vi "Main.vi"(11 "Module Admin":refnum<class "Delacor_lib_QMH_Module Admin.lvclass">) -> ()   [LabVIEW 2020, in "Aqcisition.lvlib"]
doc: "This template is based off of the Queued Message Handler design pattern and the Queued Message Handler project template that ships with LabVIEW.\n\nThe main difference is that the queue is private to this module and communication between modules is performed via Broadcast and Request events.\n\nRequest events are wrapped in public API methods and are handled in the Event Handling Loop (EHL) of this VI. Any module can register for Broadcast events sent by this module. The EHL generates messages based on user interface actions.\n\nThe Message Handling Loop (MHL) processes messages generated by the EHL, or by other messages. The messages are string values, so new messages can be added easily to the Message Cases case structure in the MHL. Each message cluster can also provide an optional value for Message Data, which is a variant that can be converted to whatever message-specific data is required.\n_____\nBased on Delacor QMH Project Template 6.0.0.89."
uses:
  Aqcisition.lvlib
  <vilib>/Delacor/Delacor QMH/Libraries/Module Admin_class/Delacor_lib_QMH_Module Admin.lvclass
  Module Data--cluster.ctl
  Analog Signal Config.ctl
  Digital Signal Config.ctl
  Stop Argument--cluster.ctl
  <vilib>/Delacor/Delacor QMH/Libraries/Message Queue_class/Delacor_lib_QMH_Message Queue.lvclass/Delacor_lib_QMH_Message Queue.ctl
  <vilib>/Delacor/Delacor QMH/Libraries/Module Admin_class/Delacor_lib_QMH_Module Admin.lvclass/Delacor_lib_QMH_Module Admin.ctl
  Start Adqcisition Argument--cluster.ctl
  Stop Adqcisition Argument--cluster.ctl
  Set AQ Parameters Argument--cluster.ctl
  <vilib>/Utility/miscctls.llb/LVPointTypeDef.ctl
  <vilib>/DAQmx/read.llb/DAQmx Read (Digital 1D U8 NChan 1Samp).vi
  <vilib>/DAQmx/read.llb/DAQmx Read (Analog 1D Wfm NChan NSamp).vi
  <vilib>/Delacor/Delacor QMH/Libraries/Message Queue_class/Delacor_lib_QMH_Enqueue Message (Single).vi
  <vilib>/Delacor/Delacor QMH/Libraries/Module Admin_class/Delacor_lib_QMH_Get External Launch.vi
  <vilib>/DAQmx/miscellaneous.llb/DAQmx Fill In Error Info.vi
  <vilib>/Utility/error.llb/Error Cluster From Error Code.vi
  <vilib>/ErrorRing/Error Ring.xnode
  <vilib>/Delacor/Delacor QMH/Libraries/Message Queue_class/Delacor_lib_QMH_Message Queue.lvclass
panel:
  out "error out":errorcluster
  out "Status":string
types:
  T1 = typedef "Aqcisition.lvlib/Request Events--cluster.ctl" = cluster{"Stop Module":refnum<user-event>, "Show Panel":refnum<user-event>, "Hide Panel":refnum<user-event>, "Get Module Execution Status":refnum<user-event>, "Show Diagram":refnum<user-event>, "Start Adqcisition":refnum<user-event>, "Stop Adqcisition":refnum<user-event>, "Wake Up Helper Loop":refnum<user-event>, "Put HL to Sleep":refnum<user-event>, "Set AQ Parameters":refnum<user-event>, "Wake up Digital Loop":refnum<user-event>}
  T2 = typedef "Aqcisition.lvlib/Module Data--cluster.ctl" = cluster{"Status":string, "Señal Analogica":T3, "Señal Digital":T4}
  T3 = typedef "Analog Signal Config.ctl" = cluster{"Canal/Canales":string, "Canal":tag, "Canales":tag[], "Frecuencia de muestreo":i32, "Numero de muestras":i32, "Tiempo de AQ":dbl}
  T4 = typedef "Digital Signal Config.ctl" = cluster{"Puertos/Pines":string, "Puerto":tag, "Pines":tag[], "Tiempo de AQ":dbl, "Tiempo entre AQ":dbl}
  T5 = enum32{"invalid lock state", "Not Locked", "Locked (No Password)", "Password-protected"}
  T6 = typedef "Aqcisition.lvlib/Stop Argument--cluster.ctl" = cluster{"Origin":string, "Exit via Stop Module Req?":bool, "Wait for Module to stop?":bool}
  T7 = typedef "Aqcisition.lvlib/Start Adqcisition Argument--cluster.ctl" = cluster{"Boolean":bool}
  T8 = typedef "Aqcisition.lvlib/Stop Adqcisition Argument--cluster.ctl" = cluster{"Boolean":bool}
  T9 = typedef "Aqcisition.lvlib/Set AQ Parameters Argument--cluster.ctl" = cluster{"Señal Analogica":T3, "Señal Digital":T4}
  T10 = typedef "LVPointTypeDef.ctl" = cluster{"Horizontal":i16, "Vertical":i16}
  T11 = enum32{"Invalid", "Standard", "Closed", "Hidden", "Minimized", "Maximized"}
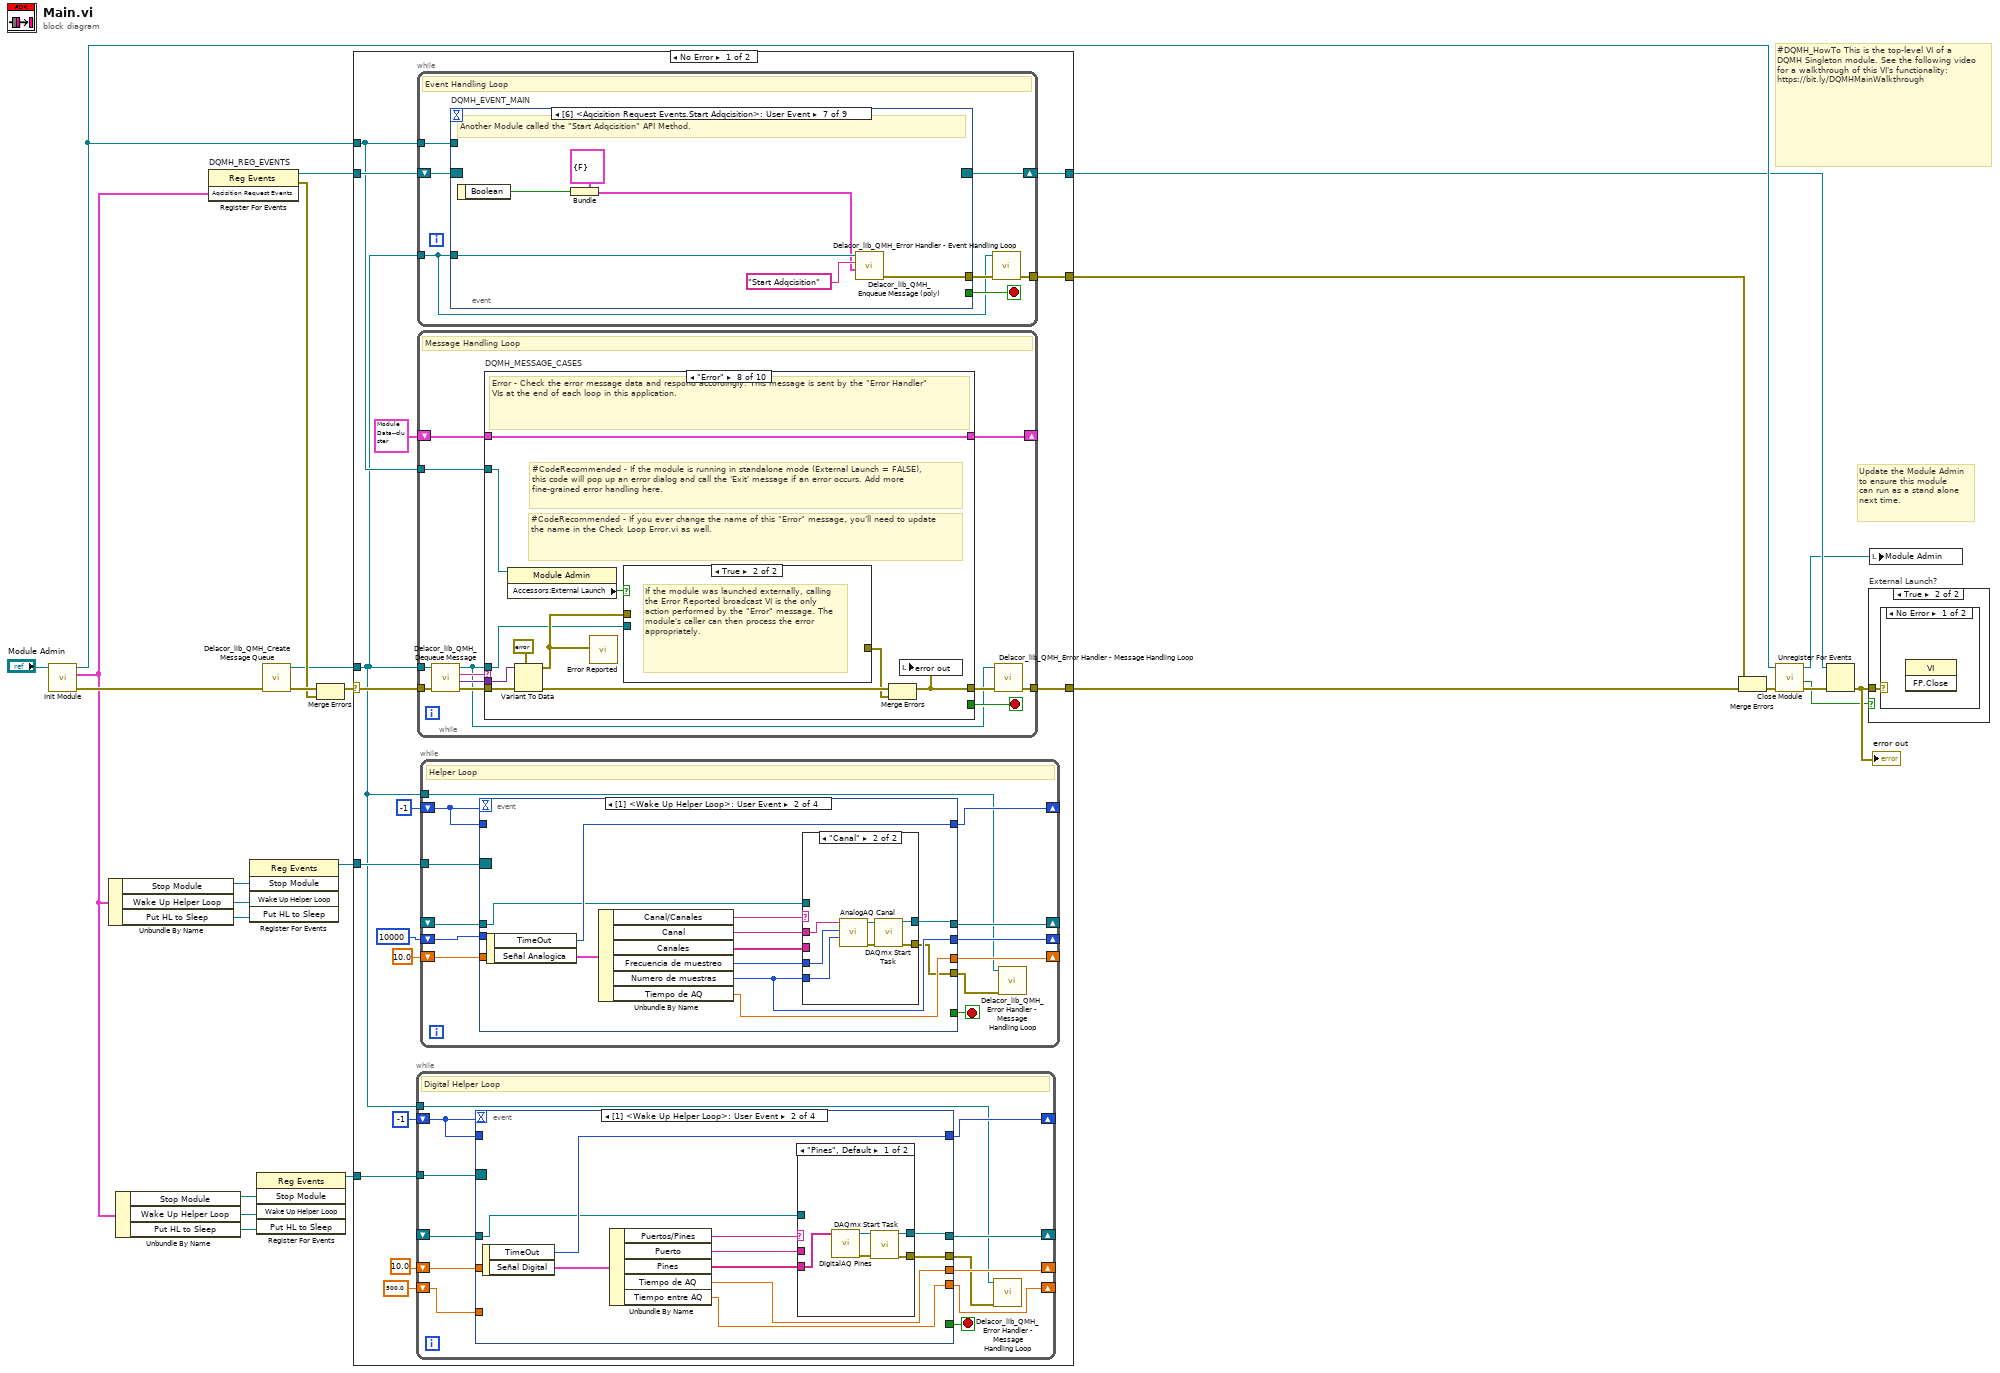
[diagram p0: block diagram]
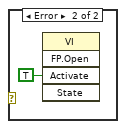
[diagram p3: hidden frame]
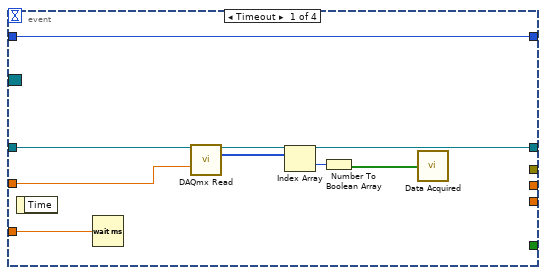
[diagram p4: hidden frame]
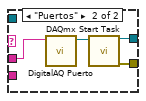
[diagram p5: hidden frame]
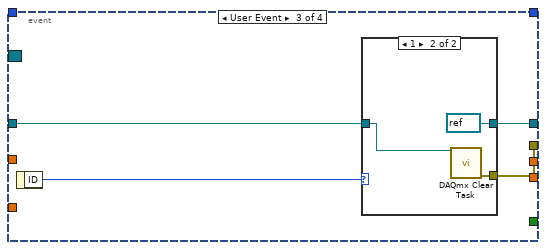
[diagram p6: hidden frame]
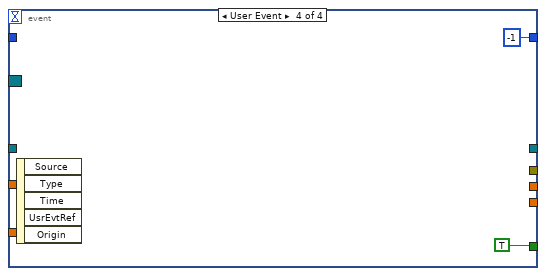
[diagram p8: hidden frame]
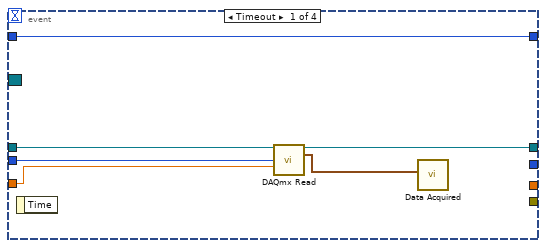
[diagram p9: hidden frame]
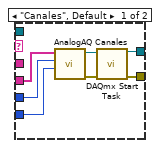
[diagram p10: hidden frame]
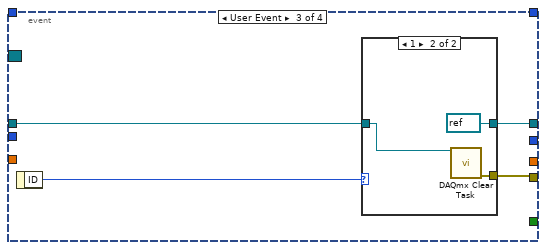
[diagram p11: hidden frame]
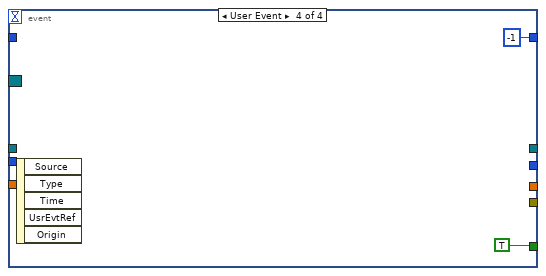
[diagram p13: hidden frame]
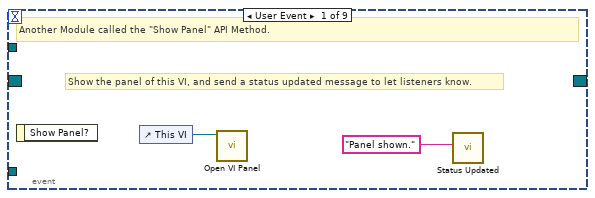
[diagram p14: hidden frame]
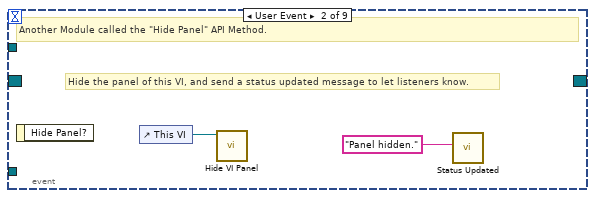
[diagram p15: hidden frame]
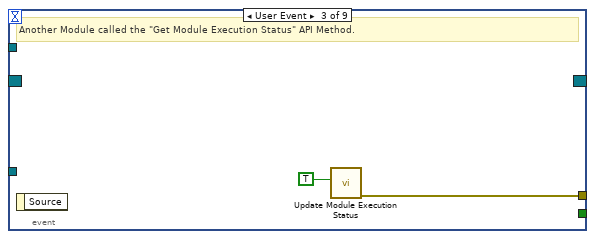
[diagram p16: hidden frame]
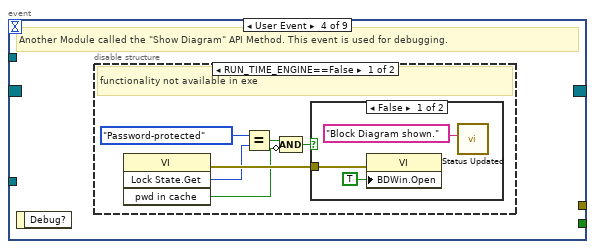
[diagram p17: hidden frame]
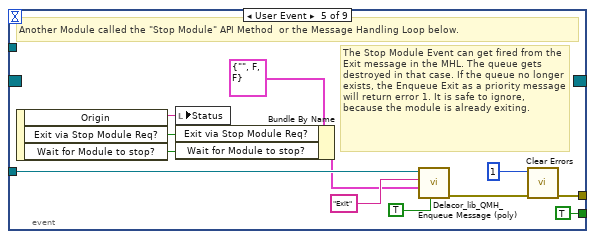
[diagram p20: hidden frame]
diagram:
  # "#DQMH_HowTo This is the top-level VI of a DQMH Singleton module. See the following video for a walkthrough of this VI's functionality: https://bit.ly/DQMHMainWalkthrough"
  # "Update the Module Admin to ensure this module can run as a stand alone next time."
  n1 = call "Init Module.vi"("Singleton Module Admin in"="Module Admin") -> ("error out"=w24:errorcluster, "Aqcisition Request Events"=w2:T1, "Singleton Module Admin out"=w16:refnum<class "Delacor_lib_QMH_Module Admin.lvclass">)  [unwired: 8 in]
  n2 = Unbundle By Name(w2) -> ("Stop Module"=w8:refnum<user-event>, "Wake Up Helper Loop"=w7:refnum<user-event>, "Put HL to Sleep"=w6:refnum<user-event>)
  n3 = Unbundle By Name(w2) -> ("Stop Module"=w3:refnum<user-event>, "Wake Up Helper Loop"=w4:refnum<user-event>, "Put HL to Sleep"=w5:refnum<user-event>)
  n4 = register-events "DQMH_REG_EVENTS"(w2) -> (reference out=w14:refnum<event-registration>, error out=w17:errorcluster)  [unwired: 2 in]
  n5 = register-events(w8, w7, w6) -> (reference out=w9:refnum<event-registration>)  [unwired: 2 in, 1 out]
  n6 = register-events(w3, w4, w5) -> (reference out=w1:refnum<event-registration>)  [unwired: 2 in, 1 out]
  n7 = call <vilib>:"Delacor_lib_QMH_Create Message Queue.vi"("error in"=w24) -> ("error out"=w19:errorcluster, "Message Queue"=w13:refnum<class "Delacor_lib_QMH_Message Queue.lvclass">)  [unwired: 9 in]
  n8 = Merge Errors(w19, w17) -> (w18:errorcluster)
  n9 = case shown="No Error" w18 {
    selector: w18 -> [w39 w315]
    tunnel: [w41 w314] -> w25
    tunnel: [w38 w320] -> w15
    tunnel: w14 -> [w36 w320]
    tunnel: w13 -> [w30 w313]
    tunnel: [w40 _] -> w22
    tunnel: w16 -> [w31 w316]
    tunnel: w9 -> [w34 _]
    tunnel: w1 -> [w29 _]
    frame No Error {
      n10 = while {
        shift-right: [w52] -> _
        shift-left: -1 ("TimeOut") -> [w53]
        tunnel: w29 -> [w51]
        shift-right: [w49] -> _
        shift-left: _ -> [w50]
        shift-right: [w48] -> _
        shift-left: 10.0 -> [w47]
        tunnel: w30 -> [w44]
        shift-right: [w43] -> _
        shift-left: 500.0 ("Tiempo entre AQ") -> [w42]
        stop <- w46 stop-if-true
        # "Digital Helper Loop"
        n11 = event shown="[1] <Wake Up Helper Loop>: User Event" {
          selector: w51 -> [_ _ _ _]
          dyn-events: _ -> [_ _ _ _]
          timeout: w53 -> [_ _ _ _]
          tunnel: w53 -> [w61 _ _ _]
          tunnel: [w61 w71 _ -1 ("TimeOut")] -> w52
          tunnel: w50 -> [w60 w66 w84 _]
          tunnel: [w59 w65 w83 _] -> w49
          tunnel: [_ w63 _ _] -> w48
          tunnel: w47 -> [w58 _ _ _]
          tunnel: [_ _ _ TRUE] -> w46
          tunnel: [_ w64 w81 _] -> w45
          tunnel: [_ w62 _ _] -> w43
          tunnel: w42 -> [w54 _ _ _]
          event Timeout {
            n12 = event-data() -> ()  [unwired: 1 in, 1 out]
            n13 = Wait (ms)(milliseconds to wait=w54) -> ()  [unwired: 1 out]
            n14 = call-poly <vilib>:"DAQmx Read.vi"("task/channels in"=w60, "timeout"=w58) -> ("task out"=w59:refnum<k21>, "data"=w57:u8[])  [unwired: 11 in, 1 out]
            n15 = Index Array(array=w57) -> (element=w56:u8)  [unwired: 1 in]
            n16 = Number To Boolean Array(number=w56) -> (Boolean array=w55:bool[])
            n17 = call "Data Acquired.vi"("Digital"=w55) -> ()  [unwired: 10 in, 1 out]
          }
          event User Event {
            n18 = event-data() -> ("TimeOut"=w71:i32, "Señal Digital"=w70:T4)  [unwired: 1 in]
            n19 = Unbundle By Name(w70) -> ("Puertos/Pines"=w69:string, "Puerto"=w68:tag, "Pines"=w67:tag[], "Tiempo de AQ"=w63:dbl, "Tiempo entre AQ"=w62:dbl)
            n20 = case shown="\"Pines\", Default" w69 {
              tunnel: w68 -> [_ w78]
              tunnel: w67 -> [w72 _]
              tunnel: w66 -> [_ _]
              tunnel: [w76 w80] -> w65
              tunnel: [w75 w79] -> w64
              frame "Pines", Default {
                n21 = call "DigitalAQ Pines.vi"("Array"=w72) -> ("error out"=w73:errorcluster, "Classic DAQmx Task Name"=w74:refnum<k21>)  [unwired: 9 in]
                n22 = call <vilib>:"DAQmx Start Task.vi"("task/channels in"=w74, "error in"=w73) -> ("task out"=w76:refnum<k21>, "error out"=w75:errorcluster)  [unwired: 12 in]
              }
              frame "Puertos" {
                n23 = call "DigitalAQ Puerto.vi"("DAQmx Board Name"=w78) -> ("Classic DAQmx Task Name"=w77:refnum<k21>)  [unwired: 9 in, 1 out]
                n24 = call <vilib>:"DAQmx Start Task.vi"("task/channels in"=w77) -> ("task out"=w80:refnum<k21>, "error out"=w79:errorcluster)  [unwired: 13 in]
              }
            }
          }
          event User Event {
            n25 = event-data() -> ("ID"=w82:i32)  [unwired: 1 in]
            n26 = case shown="1" w82 {
              tunnel: w84 -> [w85 w88]
              tunnel: [w85 refnum<k21> refnum ("task out")] -> w83
              tunnel: [_ w86] -> w81
              frame 0, Default {
              }
              frame 1 {
                n27 = call <vilib>:"DAQmx Clear Task.vi"("task in"=w88) -> ("error out"=w86:errorcluster)  [unwired: 14 in]
              }
            }
          }
          event User Event {
            n28 = event-data() -> ()  [unwired: 1 in, 5 out]
          }
        }
        n29 = call-dynamic "Delacor_lib_QMH_Error Handler - Message Handling Loop.vi"("error in"=w45, "Message Queue in"=w44) -> ()  [unwired: 8 in, 2 out]
      }
      n30 = while {
        tunnel: w30 -> [w144]
        shift-right: [w147] -> w38
        shift-left: w36 -> [w148]
        tunnel: [w149] -> w40
        tunnel: w31 -> [w145]
        stop <- w146 stop-if-true
        # "Event Handling Loop"
        n31 = event "DQMH_EVENT_MAIN" shown="[6] <Aqcisition Request Events.Start Adqcisition>: User Event" {
          selector: w148 -> [_ _ _ _ _ _ _ _ _]
          dyn-events: [_ _ _ _ _ _ _ _ _] -> w147
          timeout: _ -> [_ _ _ _ _ _ _ _ _]
          tunnel: [_ _ _ _ TRUE ("Discard?") _ _ _ _] -> w146
          tunnel: w144 -> [_ _ _ _ w173 w180 w193 w199 w206]
          tunnel: [_ _ w156 _ w176 w182 w188 w194 w200] -> w150
          tunnel: w145 -> [_ _ _ _ _ w179 _ _ _]
          event User Event {
            # "Show the panel of this VI, and send a status updated message to let listeners know."
            # "Another Module called the \"Show Panel\" API Method."
            n32 = event-data() -> ()  [unwired: 1 in, 1 out]
            n33 = control-ref of="This VI"() -> (w152:refnum<vi>)
            n34 = call "Open VI Panel.vi"("VI"=w152) -> ()  [unwired: 10 in, 1 out]
            n35 = call "Status Updated.vi"("Status"="Panel shown." ("format string")) -> ()  [unwired: 10 in, 1 out]
          }
          event User Event {
            # "Hide the panel of this VI, and send a status updated message to let listeners know."
            # "Another Module called the \"Hide Panel\" API Method."
            n36 = event-data() -> ()  [unwired: 1 in, 1 out]
            n37 = control-ref of="This VI"() -> (w154:refnum<vi>)
            n38 = call "Hide VI Panel.vi"("VI"=w154) -> ()  [unwired: 10 in, 1 out]
            n39 = call "Status Updated.vi"("Status"="Panel hidden." ("format string")) -> ()  [unwired: 10 in, 1 out]
          }
          event User Event {
            # "Another Module called the \"Get Module Execution Status\" API Method."
            n40 = event-data() -> ()  [unwired: 1 in, 1 out]
            n41 = call "Update Module Execution Status.vi"("Running?"=TRUE) -> ("error out"=w156:errorcluster)  [unwired: 10 in]
          }
          event User Event {
            # "Another Module called the \"Show Diagram\" API Method. This event is used for debugging."
            n42 = event-data() -> ()  [unwired: 1 in, 1 out]
            n43 = disable-structure shown="RUN_TIME_ENGINE==False" {
              frame condition #0 (active) {
                # "functionality not available in exe"
                n44 = invoke class="VI" method="Lock State.Get"() -> (error out=w162:errorcluster, "Get Lock State"=w161:T5, "pwd in cache"=w158:bool)  [unwired: 4 in, 1 out]
                n45 = Equal?(x=T5."Password-protected", y=w161) -> (x = y?=w159:bool)
                n46 = Compound Arithmetic op=AND(w159, invert w158) -> (w157:bool)
                n47 = case shown="False" w157 {
                  tunnel: w162 -> [w165 _]
                  frame False {
                    n48 = property class="VI"(error in=w165, "BDWin.Open"=TRUE ("Block Diagram Window:Open")) -> ()  [unwired: 1 in, 2 out]
                    n49 = call "Status Updated.vi"("Status"="Block Diagram shown." ("format string")) -> ()  [unwired: 10 in, 1 out]
                  }
                  frame True {
                    # "Password-protected VI, and the password is not in the cache. Do not show the diagram."
                  }
                }
              }
              frame condition #1 {
              }
            }
          }
          event User Event {
            # "The Stop Module Event can get fired from the Exit message in the MHL. The queue gets destroyed in that case. If the queue no longer exists, the Enqueue Exit as a priority message will return error 1. It is safe to ignore, because the module is already exiting."
            # "Another Module called the \"Stop Module\" API Method  or the Message Handling Loop below."
            n50 = event-data() -> ("Origin"=w172:string, "Exit via Stop Module Req?"=w168:bool, "Wait for Module to stop?"=w167:bool)  [unwired: 1 in]
            n51 = local write "Status"(w172) -> ()
            n52 = Bundle By Name(cluster=T6 {"Origin"="", "Exit via Stop Module Req?"=FALSE, "Wait for Module to stop?"=FALSE} ("Stop Argument"), "Exit via Stop Module Req?"=w168, "Wait for Module to stop?"=w167) -> (w166:T6)
            n53 = call-poly <vilib>:"Delacor_lib_QMH_Enqueue Message (poly).vi"("Priority Message? (F)"=TRUE, "Message Data"=w166, "Message"="Exit", "Message Queue in"=w173) -> ("error out"=w177:errorcluster)  [unwired: 6 in, 1 out]
            n54 = call <vilib>:"Clear Errors.vi"("error in (no error)"=w177, "specific error code to clear (0: all)"=1) -> ("error out"=w176:errorcluster)  [unwired: 4 in, 1 out]
          }
          event Panel Close? {
            w181 = TRUE  # Discard the event, the MHL is responsible for closing and stopping this VI.
            # "Hide the panel or send the 'Exit' message if the user clicks the 'X' on the module main VI panel."
            n55 = event-data() -> ()  [unwired: 1 in, 1 out]
            n56 = property class="Module Admin"(reference=w179) -> ("Accessors:External Launch"=w178:bool)  [unwired: 1 in, 2 out]
            n57 = case shown="False" w178 {
              tunnel: w180 -> [_ w186]
              tunnel: [_ w187] -> w182
              frame True {
                # "If externally launched, clicking the 'X' hides the panel, but doesn't close it."
                n58 = control-ref of="This VI"() -> (w183:refnum<vi>)
                n59 = call "Hide VI Panel.vi"("VI"=w183) -> ()  [unwired: 10 in, 1 out]
              }
              frame False {
                # "If run as a stand-alone VI, clicking the panel 'X' stops the VI."
                n60 = call-poly <vilib>:"Delacor_lib_QMH_Enqueue Message (poly).vi"("Priority Message? (F)"=TRUE, "Message"="Exit", "Message Queue in"=w186) -> ("error out"=w187:errorcluster)  [unwired: 7 in, 1 out]
              }
            }
            n61 = event-data("Discard?"=w181) -> ()  [unwired: 1 in, 1 out]
          }
          event User Event {
            # "Another Module called the \"Start Adqcisition\" API Method."
            n62 = event-data() -> ("Boolean"=w189:bool)  [unwired: 1 in]
            n63 = Bundle(cluster=T7 {"Boolean"=FALSE} ("Start Adqcisition Argument"), "Boolean"=w189) -> (w190:T7)
            n64 = call-poly <vilib>:"Delacor_lib_QMH_Enqueue Message (poly).vi"("Message Data"=w190, "Message"="Start Adqcisition", "Message Queue in"=w193) -> ("error out"=w188:errorcluster)  [unwired: 7 in, 1 out]
          }
          event User Event {
            # "Another Module called the \"Stop Adqcisition\" API Method."
            n65 = event-data() -> ("Boolean"=w195:bool)  [unwired: 1 in]
            n66 = Bundle(cluster=T8 {"Boolean"=FALSE} ("Stop Adqcisition Argument"), "Boolean"=w195) -> (w196:T8)
            n67 = call-poly <vilib>:"Delacor_lib_QMH_Enqueue Message (poly).vi"("Message Data"=w196, "Message"="Stop Adqcisition", "Message Queue in"=w199) -> ("error out"=w194:errorcluster)  [unwired: 7 in, 1 out]
          }
          event User Event {
            # "Another Module called the \"Set AQ Parameters\" API Method."
            n68 = event-data() -> ("Señal Analogica"=w202:T3, "Señal Digital"=w201:T4)  [unwired: 1 in]
            n69 = Bundle(cluster=T9 {"Señal Analogica"={"Canal/Canales"="", "Canal"="DAQSim1", "Canales"=[], "Frecuencia de muestreo"=1000, "Numero de muestras"=1000, "Tiempo de AQ"=0.0}, "Señal Digital"={"Puertos/Pines"="", "Puerto"="DAQSim1", "Pines"=[], "Tiempo de AQ"=0.0, "Tiempo entre AQ"=0.0}} ("Set AQ Parameters Argument"), "Señal Analogica"=w202, "Señal Digital"=w201) -> (w203:T9)
            n70 = call-poly <vilib>:"Delacor_lib_QMH_Enqueue Message (poly).vi"("Message Data"=w203, "Message"="Set AQ Parameters", "Message Queue in"=w206) -> ("error out"=w200:errorcluster)  [unwired: 7 in, 1 out]
          }
        }
        n71 = call-dynamic "Delacor_lib_QMH_Error Handler - Event Handling Loop.vi"("error in"=w150, "Message Queue in"=w144) -> ("dup error in"=w149:errorcluster)  [unwired: 8 in, 1 out]
      }
      n72 = while {
        tunnel: w30 -> [w209]
        shift-right: [w213] -> _
        shift-left: T2 {"Status"="", "Señal Analogica"={"Canal/Canales"="Canal", "Canal"="DAQSim1", "Canales"=[], "Frecuencia de muestreo"=1000, "Numero de muestras"=1000, "Tiempo de AQ"=10.0}, "Señal Digital"={"Puertos/Pines"="Puertos", "Puerto"="DAQSim1", "Pines"=[], "Tiempo de AQ"=0.0, "Tiempo entre AQ"=0.0}} ("Data Cluster") -> [w214]
        tunnel: w39 -> [w217]
        tunnel: [w215] -> w41
        tunnel: w31 -> [w207]
        stop <- w212 stop-if-true
        # "Message Handling Loop"
        n73 = call-dynamic "Delacor_lib_QMH_Dequeue Message.vi"("error in"=w217, "Message Queue in"=w209) -> ("error out"=w216:errorcluster, "Message Data"=w210:variant, "Message"=w211:string, "Message Queue out"=w208:refnum<class "Delacor_lib_QMH_Message Queue.lvclass">)  [unwired: 6 in]
        n74 = case "DQMH_MESSAGE_CASES" shown="\"Error\"" w211 {
          selector: w211 -> [_ _ _ _ _ _ _ _ _ w300]
          tunnel: w208 -> [_ _ _ _ _ _ _ w270 w292 _]
          tunnel: w216 -> [w236 w240 w249 w252 w262 w265 w267 w277 w298 w302]
          tunnel: [w234 w240 w248 w251 w261 w264 w267 w273 w295 w303] -> w218
          tunnel: w214 -> [w225 w239 w244 w253 w256 w263 w266 w272 w291 w301]
          tunnel: [w224 w239 w244 w253 w257 w263 w266 w272 w291 w301] -> w213
          tunnel: [_ _ _ _ _ _ _ _ w290 _] -> w212
          tunnel: w210 -> [_ _ w247 _ w260 _ _ w271 w289 _]
          tunnel: w207 -> [w226 _ _ _ _ _ _ w269 w284 _]
          frame "Initialize" {
            w220 = "Initial Message" ("Initial Message")
            # "#CodeNeeded - Initialize the appearance of the front panel."
            # "#CodeNeeded - Initialize your state data here."
            # "Initialize - Any operation that needs to be done before the module can receive messages. Synchronize Caller Events.vi will inform Start Module.vi that the module has launched and is ready to receive messages. Module Did Init.vi will broadcast that the module initialized."
            n75 = call "Synchronize Caller Events.vi"("error in (no error)"=w236, "Singleton Module Admin in"=w226) -> ("error out"=w235:errorcluster, "Singleton Module Admin out"=w221:refnum<class "Delacor_lib_QMH_Module Admin.lvclass">)  [unwired: 8 in]
            n76 = property class="Module Admin"(reference=w221) -> ("Accessors:External Launch"=w230:bool)  [unwired: 1 in, 2 out]
            n77 = Select(t=T11."Hidden" ("State"), s=w230, f=T11."Standard" ("State")) -> (s? t:f=w227:T11)
            n78 = call "Module Name--constant.vi"() -> ("Module Name"=w233:string)  [unwired: 11 in]
            n79 = property class="VI"("Front Panel.Title"=w233) -> (reference out=w232:refnum<vi>, error out=w238:errorcluster)  [unwired: 2 in]
            n80 = call "Module Name--constant.vi"() -> ("Module Name"=w222:string)  [unwired: 11 in]
            n81 = invoke class="VI" method="FP.Open"(reference=w232, error in=w238, "State"=w227) -> (reference out=w231:refnum<vi>, error out=w237:errorcluster)  [unwired: 2 in, 3 out]
            n82 = Bundle By Name(cluster=w225, "Status"=w220) -> (w224:T2)
            n83 = call "Module Did Init.vi"("error in (no error)"=w235, "Initialized?"=TRUE, "Origin"=w222) -> ("error out"=w234:errorcluster)  [unwired: 8 in]
            n84 = invoke class="VI" method="FP.Center"(reference=w231, error in=w237) -> ()  [unwired: 1 in, 3 out]
            n85 = property on="Pane" class="Pane"("Origin"=T10 {"Horizontal"=0, "Vertical"=0}) -> ()  [unwired: 2 in, 2 out]
            "Status" <- w220
          }
          frame "---Module Specific---" {
            # "Separator -- The following cases handle messages specific to this Module."
          }
          frame "Start Adqcisition" {
            # "Start AQ"
            n86 = Variant To Data(error in=w249, type=T7 {"Boolean"=FALSE} ("Start Adqcisition Argument"), Variant=w247) -> (data=w245:T7, error out=w248:errorcluster)
            n87 = Unbundle By Name(w245) -> ()  [unwired: 1 out]
            n88 = Unbundle By Name(w244) -> ("Señal Analogica"=w243:T3, "Señal Digital"=w242:T4)
            n89 = call "Wake Up Helper Loop.vi"("TimeOut"=0, "Señal Digital"=w242, "Señal Analogica"=w243) -> ()  [unwired: 8 in, 1 out]
          }
          frame "Stop Adqcisition" {
            # "Stop AQ"
            n90 = call "Put HL to Sleep.vi"("error in"=w252, "ID"=1) -> ("error out"=w251:errorcluster)  [unwired: 9 in]
          }
          frame "Set AQ Parameters" {
            # "It will indicate what are we going to see"
            n91 = Variant To Data(error in=w262, type=T9 {"Señal Analogica"={"Canal/Canales"="", "Canal"="DAQSim1", "Canales"=[], "Frecuencia de muestreo"=1000, "Numero de muestras"=1000, "Tiempo de AQ"=0.0}, "Señal Digital"={"Puertos/Pines"="", "Puerto"="DAQSim1", "Pines"=[], "Tiempo de AQ"=0.0, "Tiempo entre AQ"=0.0}} ("Set AQ Parameters Argument"), Variant=w260) -> (data=w258:T9, error out=w261:errorcluster)
            n92 = Unbundle By Name(w258) -> ("Señal Analogica"=w255:T3, "Señal Digital"=w254:T4)
            n93 = Bundle By Name(cluster=w256, "Señal Analogica"=w255, "Señal Digital"=w254) -> (w257:T2)
          }
          frame "---Copy This Frame---" {
            # "Duplicate this frame when creating new messages.  Change this comment in the duplicated frame to describe this message."
            n94 = Merge Errors(w265) -> (w264:errorcluster)
          }
          frame "---Exit and Error Handling---" {
            # "Separator - The following cases handle errors and exit messages."
          }
          frame "Error" {
            # "#CodeRecommended - If you ever change the name of this \"Error\" message, you'll need to update the name in the Check Loop Error.vi as well."
            # "#CodeRecommended - If the module is running in standalone mode (External Launch = FALSE), this code will pop up an error dialog and call the 'Exit' message if an error occurs. Add more fine-grained error handling here."
            # "Error - Check the error message data and respond accordingly. This message is sent by the \"Error Handler\" VIs at the end of each loop in this application."
            n95 = property class="Module Admin"(reference=w269) -> ("Accessors:External Launch"=w268:bool)  [unwired: 1 in, 2 out]
            n96 = Variant To Data(error in=w277, type=errorcluster {"status"=FALSE, "code"=0, "source"=""} ("error constant"), Variant=w271) -> (data=w278:errorcluster, error out=w275:errorcluster)
            n97 = call "Error Reported.vi"("Error"=w278) -> ()  [unwired: 10 in, 1 out]
            n98 = case shown="True" w268 {
              tunnel: [w283 _] -> w274
              tunnel: w270 -> [w281 _]
              tunnel: w278 -> [w282 _]
              frame False {
                # "If the module is running standalone, then pop up an error dialog and call the \"Exit\" message."
                n99 = call <vilib>:"Simple Error Handler.vi"("error in (no error)"=w282) -> ()  [unwired: 4 in, 5 out]
                n100 = call-poly <vilib>:"Delacor_lib_QMH_Enqueue Message (poly).vi"("Priority Message? (F)"=TRUE, "Message"="Exit", "Message Queue in"=w281) -> ("error out"=w283:errorcluster)  [unwired: 7 in, 1 out]
              }
              frame True {
                # "If the module was launched externally, calling the Error Reported broadcast VI is the only action performed by the \"Error\" message. The module's caller can then process the error appropriately."
              }
            }
            n101 = Merge Errors(w275, w274) -> (w273:errorcluster)
            n102 = local write "error out"(w273) -> ()
          }
          frame "Exit" {
            w288 = 91  # 91: not all Exit messages will have an argument
            w290 = TRUE  # Stop the VI
            # "Release the message queue reference"
            # "#CodeNeeded - Add any required cleanup code here"
            # "Exit - Exit the application."
            n103 = Variant To Data(error in=w298, type=T6 {"Origin"="", "Exit via Stop Module Req?"=FALSE, "Wait for Module to stop?"=FALSE} ("Stop Argument"), Variant=w289) -> (data=w286:T6, error out=w294:errorcluster)
            n104 = call <vilib>:"Clear Errors.vi"("error in (no error)"=w294, "specific error code to clear (0: all)"=w288) -> ("error out"=w297:errorcluster)  [unwired: 4 in, 1 out]
            n105 = control-ref of="This VI"() -> (w285:refnum<vi>)
            n106 = call-dynamic "Delacor_lib_QMH_Release Message Queue.vi"("error in"=w297, "Message Queue"=w292) -> ("error out"=w296:errorcluster)  [unwired: 9 in]
            n107 = call "Handle Exit.vi"("Stop Argument"=w286, "Admin in"=w284, "VI reference"=w285) -> ("error out"=w293:errorcluster)  [unwired: 7 in, 1 out]
            n108 = Merge Errors(w296, w293) -> (w295:errorcluster)
          }
          frame Default {
            # "'Default' case only runs if there is a message that isn't defined in any of the other cases.  Output a programming error."
            n109 = call "Module Name--constant.vi"() -> ("Module Name"=w299:string)  [unwired: 11 in]
            n110 = xnode "Error Ring"("parameter 0"=w300, "parameter 1"=w299) -> ("error out"=w304:errorcluster)
            n111 = Merge Errors(w302, w304) -> (w303:errorcluster)
          }
        }
        n112 = call-dynamic "Delacor_lib_QMH_Error Handler - Message Handling Loop.vi"("error in"=w218, "Message Queue in"=w208) -> ("dup error in"=w215:errorcluster)  [unwired: 8 in, 1 out]
      }
      n113 = while {
        shift-right: [w101] -> _
        shift-left: -1 -> [w102]
        tunnel: w34 -> [w100]
        shift-right: [w98] -> _
        shift-left: _ -> [w99]
        shift-right: [w97] -> _
        shift-left: 10.0 ("Tiempo de AQ") -> [w96]
        shift-right: [w95] -> _
        shift-left: 10000 ("Numero de muestras") -> [w94]
        tunnel: w30 -> [w91]
        stop <- w93 stop-if-true
        # "Helper Loop"
        n114 = event shown="[1] <Wake Up Helper Loop>: User Event" {
          selector: w100 -> [_ _ _ _]
          dyn-events: _ -> [_ _ _ _]
          timeout: w102 -> [_ _ _ _]
          tunnel: w102 -> [w108 _ _ _]
          tunnel: [w108 w119 _ -1 ("TimeOut")] -> w101
          tunnel: w99 -> [w107 w113 w137 _]
          tunnel: [w106 w112 w136 _] -> w98
          tunnel: [_ w111 _ _] -> w97
          tunnel: w96 -> [w105 _ _ _]
          tunnel: [_ w110 _ _] -> w95
          tunnel: w94 -> [w104 _ _ _]
          tunnel: [_ _ _ TRUE] -> w93
          tunnel: [_ w109 w134 _] -> w92
          event Timeout {
            n115 = event-data() -> ()  [unwired: 1 in, 1 out]
            n116 = call-poly <vilib>:"DAQmx Read.vi"("task/channels in"=w107, "number of samples per channel"=w104, "timeout"=w105) -> ("task out"=w106:refnum<k21>, "data"=w103:waveform(dbl)[])  [unwired: 10 in, 1 out]
            n117 = call "Data Acquired.vi"("Analog"=w103) -> ()  [unwired: 10 in, 1 out]
          }
          event User Event {
            n118 = event-data() -> ("TimeOut"=w119:i32, "Señal Analogica"=w118:T3)  [unwired: 1 in]
            n119 = Unbundle By Name(w118) -> ("Canal/Canales"=w117:string, "Canal"=w116:tag, "Canales"=w115:tag[], "Frecuencia de muestreo"=w114:i32, "Numero de muestras"=w110:i32, "Tiempo de AQ"=w111:dbl)
            n120 = case shown="\"Canal\"" w117 {
              tunnel: w116 -> [_ w130]
              tunnel: w115 -> [w123 _]
              tunnel: w114 -> [w122 w129]
              tunnel: w110 -> [w121 w128]
              tunnel: w113 -> [_ _]
              tunnel: [w126 w131] -> w112
              tunnel: [w120 w127] -> w109
              frame "Canales", Default {
                n121 = call "AnalogAQ Canales.vi"("Numero de Muestras"=w121, "Frecuencia"=w122, "Canales"=w123) -> ("error out"=w125:errorcluster, "Classic DAQmx Task Name"=w124:refnum<k21>)  [unwired: 7 in]
                n122 = call <vilib>:"DAQmx Start Task.vi"("task/channels in"=w124, "error in"=w125) -> ("task out"=w126:refnum<k21>, "error out"=w120:errorcluster)  [unwired: 12 in]
              }
              frame "Canal" {
                n123 = call "AnalogAQ Canal.vi"("Numero de Muestras"=w128, "Frecuencia"=w129, "DAQmx Board Name"=w130) -> ("error out"=w132:errorcluster, "Classic DAQmx Task Name"=w133:refnum<k21>)  [unwired: 7 in]
                n124 = call <vilib>:"DAQmx Start Task.vi"("task/channels in"=w133, "error in"=w132) -> ("task out"=w131:refnum<k21>, "error out"=w127:errorcluster)  [unwired: 12 in]
              }
            }
          }
          event User Event {
            n125 = event-data() -> ("ID"=w135:i32)  [unwired: 1 in]
            n126 = case shown="1" w135 {
              tunnel: w137 -> [w138 w141]
              tunnel: [w138 refnum<k21> refnum ("task out")] -> w136
              tunnel: [_ w139] -> w134
              frame 0, Default {
              }
              frame 1 {
                n127 = call <vilib>:"DAQmx Clear Task.vi"("task in"=w141) -> ("error out"=w139:errorcluster)  [unwired: 14 in]
              }
            }
          }
          event User Event {
            n128 = event-data() -> ()  [unwired: 1 in, 5 out]
          }
        }
        n129 = call-dynamic "Delacor_lib_QMH_Error Handler - Message Handling Loop.vi"("error in"=w92, "Message Queue in"=w91) -> ()  [unwired: 8 in, 2 out]
      }
    }
    frame Error {
      # "Synchronize Caller Events.vi will inform Start Module.vi that the module has launched and will let the code calling Start Module.vi register for broadcasts and would permit the caller receive the broadcast that an error occurred at launch time."
      n130 = call-dynamic "Delacor_lib_QMH_Release Message Queue.vi"("error in"=w315, "Message Queue"=w313) -> ("error out"=w314:errorcluster)  [unwired: 9 in]
      n131 = call "Synchronize Caller Events.vi"("Singleton Module Admin in"=w316) -> ("error out"=w321:errorcluster)  [unwired: 9 in, 1 out]
      n132 = call "Module Name--constant.vi"() -> ("Module Name"=w319:string)  [unwired: 11 in]
      n133 = Format Into String(format string="An error occurred during initialization. %s is no longer running.", w319) -> (resulting string=w317:string)  [unwired: 2 in, 1 out]
      n134 = Merge Errors(w314, w321) -> (w322:errorcluster)
      n135 = call "Error Reported.vi"("Additional Information"=w317, "Error"=w322) -> ()  [unwired: 9 in, 1 out]
    }
  }
  n136 = Merge Errors(w22, w25) -> (w21:errorcluster)
  n137 = call "Close Module.vi"("error in (no error)"=w21, "Module Admin in"=w16) -> ("error out"=w23:errorcluster, "External Launch"=w10:bool, "Module Admin out"=w11:refnum<class "Delacor_lib_QMH_Module Admin.lvclass">)  [unwired: 7 in]
  n138 = Unregister For Events(event registration refnum=w15, error in=w23) -> (error out=w20:errorcluster)
  "error out" <- w20
  n139 = case "External Launch?" shown="True" w10 {
    tunnel: w20 -> [_ w323]
    frame False {
    }
    frame True {
      n140 = case shown="No Error" w323 {
        frame No Error {
          n141 = invoke class="VI" method="FP.Close"() -> ()  [unwired: 3 in, 3 out]
        }
        frame Error {
          n142 = invoke class="VI" method="FP.Open"("Activate"=TRUE ("Activate?")) -> ()  [unwired: 4 in, 5 out]
        }
      }
    }
  }
  n143 = local write "Module Admin"(w11) -> ()
